vi "Trigger.vi"(11 "Menu event":refnum<user-event>) -> ()   [LabVIEW 2009]
panel:
  in  "Source":bool
  in  "Level":dbl(knob) min=-2.0 max=2.0 scale format="%0.2f"
  in  "Slope":bool
  # "-"
  # "+"
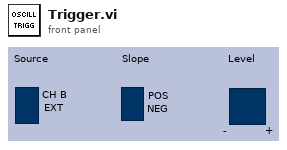
[diagram p1: front panel]
types:
  T1 = enum8{"Enabled", "Disabled", "Disabled and Grayed Out"}
  T2 = enum16{"All Elements", "Channel", "Source", "Level", "Slope", "Time Base", "Volts / Div"}
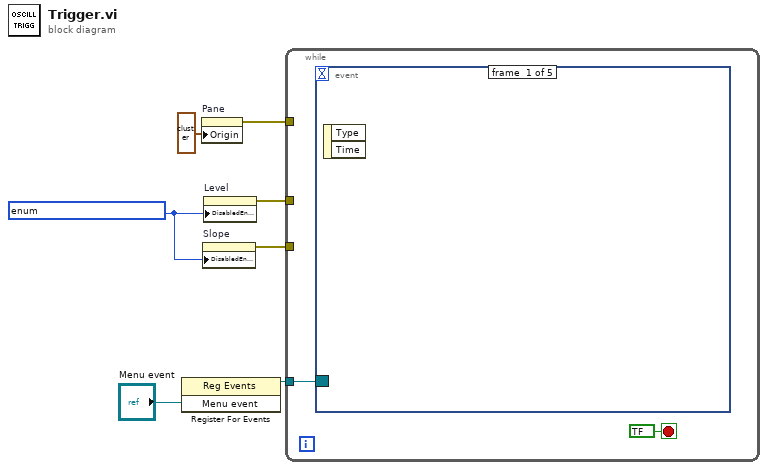
[diagram p0: block diagram]
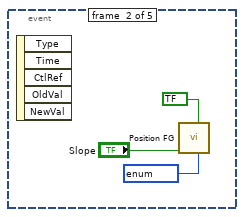
[diagram p2: hidden frame]
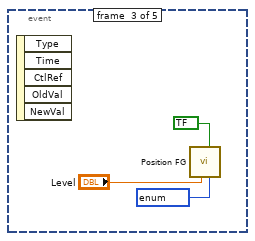
[diagram p3: hidden frame]
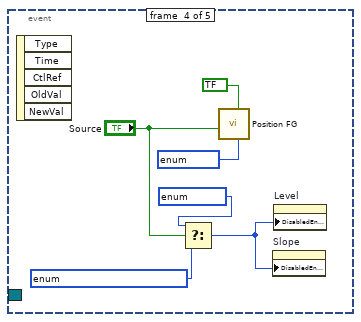
[diagram p4: hidden frame]
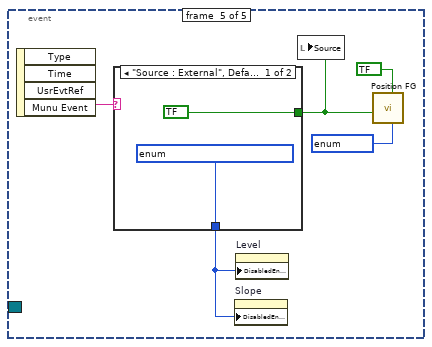
[diagram p5: hidden frame]
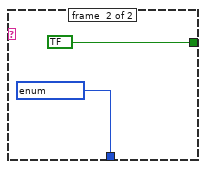
[diagram p6: hidden frame]
diagram:
  w5 = T1 ? ("Disabled")
  n1 = register-events("Menu event") -> (reference out=w7:refnum<event-registration>)  [unwired: 2 in, 1 out]
  n2 = property on="Pane" class="Pane"("Origin"=cluster{"Horizontal":i16, "Vertical":i16} ?) -> (error out=w1:errorcluster)  [unwired: 2 in, 1 out]
  n3 = property on="Slope" class="Bool (strict)"("DisabledEnum"=w5) -> (error out=w3:errorcluster)  [unwired: 2 in, 1 out]
  n4 = property on="Level" class="Knob (strict)"("DisabledEnum"=w5) -> (error out=w4:errorcluster)  [unwired: 2 in, 1 out]
  n5 = while {
    tunnel: w7 -> [w8]
    tunnel: w4 -> [_]
    tunnel: w3 -> [_]
    tunnel: w1 -> [_]
    stop <- bool ? stop-if-true
    n6 = event shown="[4] <Menu event>: User Event" {
      selector: w8 -> [_ _ _ _ _]
      dyn-events: _ -> [_ _ _ _ _]
      timeout: _ -> [_ _ _ _ _]
      event #0 {
        n7 = event-data() -> ()  [unwired: 1 in, 2 out]
      }
      event #1 {
        n8 = event-data() -> ()  [unwired: 1 in, 5 out]
        n9 = call "Position FG.vi"("Parameter"=T2 ?, "Get / Set (T=Set)"=bool ?, "Slope"="Slope") -> ()  [unwired: 8 in, 1 out]
      }
      event #2 {
        n10 = event-data() -> ()  [unwired: 1 in, 5 out]
        n11 = call "Position FG.vi"("Parameter"=T2 ?, "Get / Set (T=Set)"=bool ?, "Level"="Level") -> ()  [unwired: 8 in, 1 out]
      }
      event #3 {
        n12 = event-data() -> ()  [unwired: 1 in, 5 out]
        n13 = Select(t=T1 ? ("Disabled"), s="Source", f=T1 ? ("Disabled")) -> (s? t:f=w16:T1)
        n14 = call "Position FG.vi"("Parameter"=T2 ?, "Get / Set (T=Set)"=bool ?, "Source"="Source") -> ()  [unwired: 8 in, 1 out]
        n15 = property on="Slope" class="Bool (strict)"("DisabledEnum"=w16) -> ()  [unwired: 2 in, 2 out]
        n16 = property on="Level" class="Knob (strict)"("DisabledEnum"=w16) -> ()  [unwired: 2 in, 2 out]
      }
      event #4 {
        n17 = event-data() -> ("Munu Event"=w26:string)  [unwired: 1 in, 3 out]
        n18 = case shown="\"Source : External\", Default" w26 {
          tunnel: [T1 ? ("Disabled") T1 ? ("Disabled")] -> w25
          tunnel: [bool ? ("Source") bool ? ("Source")] -> w22
          frame #0 {
          }
          frame #1 {
          }
        }
        n19 = property on="Slope" class="Bool (strict)"("DisabledEnum"=w25) -> ()  [unwired: 2 in, 2 out]
        n20 = property on="Level" class="Knob (strict)"("DisabledEnum"=w25) -> ()  [unwired: 2 in, 2 out]
        n21 = local write "Source"(w22) -> ()
        n22 = call "Position FG.vi"("Parameter"=T2 ?, "Get / Set (T=Set)"=bool ?, "Source"=w22) -> ()  [unwired: 8 in, 1 out]
      }
    }
  }
